vi "GUID Allocator.vi"(10 "Reinit GUID (Danger!)":bool) -> (3 "New GUID":u16)   [LabVIEW 2013]
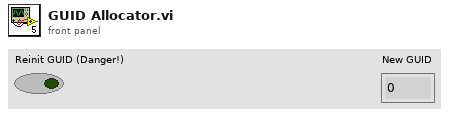
[diagram p1: front panel]
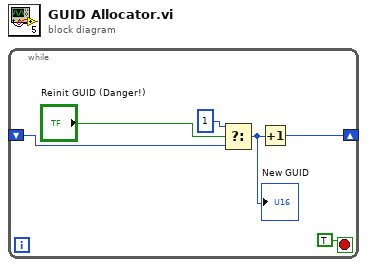
[diagram p0: block diagram]
diagram:
  n1 = while {
    shift-right: [w5] -> _
    shift-left: _ -> [w3]
    stop <- TRUE stop-if-true
    n2 = Select(t=u16 1, s="Reinit GUID (Danger!)", f=w3) -> (s? t:f=w4:u16)
    "New GUID" <- w4
    n3 = Increment(x=w4) -> (x+1=w5:u16)
  }
